vi "Sub_NMEA-LatLong.vi"(9 "lon_index":i32=4, 10 "lat_index":i32=2, 11 "str-arr_GNGGA":string[](array[string])=["", "061711.00", "3513.14928", "N", "12901.22133", "E", "1", "12", "0.52", "53.3", "M", "24.2", "M", "", "*7F"]) -> (3 "latlong":cluster{"Lat":dbl, "Long":dbl})   [LabVIEW 2019]
panel:
  out "lon":dbl
  out "lat":dbl
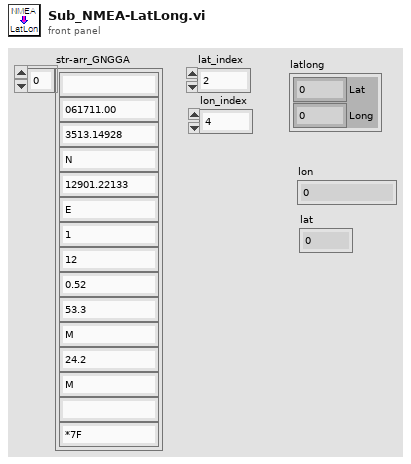
[diagram p1: front panel]
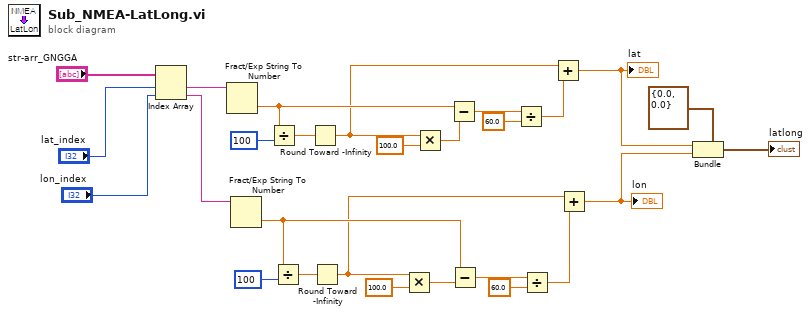
[diagram p0: block diagram]
diagram:
  n1 = Index Array(array="str-arr_GNGGA", index #1="lat_index", index #2="lon_index") -> (element #1=w14:string, element #2=w13:string)
  n2 = Fract/Exp String To Number(string=w14) -> (number=w16:dbl)  [unwired: 3 in, 1 out]
  n3 = Fract/Exp String To Number(string=w13) -> (number=w15:dbl)  [unwired: 3 in, 1 out]
  n4 = Divide(x=w16, y=100) -> (x/y=w20:dbl)
  n5 = Divide(x=w15, y=100) -> (x/y=w17:dbl)
  n6 = Round Toward -Infinity(1:w20) -> (0:w7:dbl)
  n7 = Round Toward -Infinity(1:w17) -> (0:w5:dbl)
  n8 = Multiply(x=w5, y=100.0) -> (x*y=w18:dbl)
  n9 = Multiply(x=w7, y=100.0) -> (x*y=w19:dbl)
  n10 = Subtract(x=w16, y=w19) -> (x-y=w12:dbl)
  n11 = Subtract(x=w15, y=w18) -> (x-y=w9:dbl)
  n12 = Divide(x=w12, y=60.0) -> (x/y=w8:dbl)
  n13 = Divide(x=w9, y=60.0) -> (x/y=w6:dbl)
  n14 = Add(x=w7, y=w8) -> (x+y=w4:dbl)
  "lat" <- w4
  n15 = Add(x=w5, y=w6) -> (x+y=w3:dbl)
  "lon" <- w3
  n16 = Bundle(cluster=cluster{"lat":dbl, "lon":dbl} {"lat"=0.0, "lon"=0.0} ("클러스터"), "lat"=w4, "lon"=w3) -> (→"latlong":cluster{"lat":dbl, "lon":dbl})
